vi "DUTDialog.vi"(8 "Error In":errorcluster, 11 "DUT Configuration In":T1={"Count"=1, "Wirings"=[], "Names"=[]}) -> (0 "Error Out":errorcluster, 2 "Cancelled?":bool, 3 "DUT Configuration Out":T1={"Count"=1, "Wirings"=[], "Names"=[]})   [LabVIEW 2012]
uses:
  DUTConfiguration.ctl
  driver/Public/Controls/SMUSense.ctl
  libs/LV-Utilities/LV-Utilities.lvlib
  driver/Keithley-2602.lvlib
panel:
  in  "CANCEL":bool
  in  "DONE":bool
  in  "SMU B Names":string[](array[string])
  in  "SMU B Wiring":enum16{"2-Wire", "4-Wire"}(ring)=enum."4-Wire"
  in  "SMU A Names":string[](array[string])
  in  "SMU A Wiring":enum16{"2-Wire", "4-Wire"}(ring)=enum."4-Wire"
  in  "Count":u32=1 min=1 step=1
  # "Source-Measure Unit A"
  # "Source-Measure Unit B"
  # "Names"
  # "Wiring"
  # "Names"
  # "Wiring"
  # "Number Per SMU:"
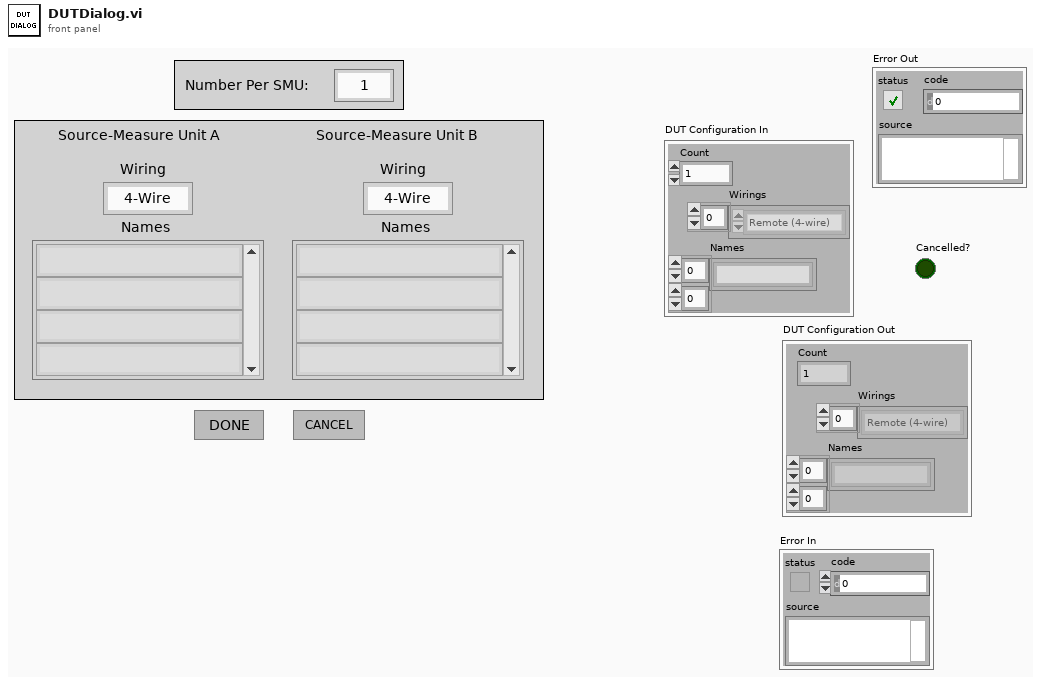
[diagram p1: front panel]
types:
  T1 = typedef "DUTConfiguration.ctl" = cluster{"Count":u32, "Wirings":T2[], "Names":string[][]}
  T2 = typedef "Keithley-2602.lvlib/SMUSense.ctl" = enum16{"Local (2-wire)", "Remote (4-wire)", "Calibration"}
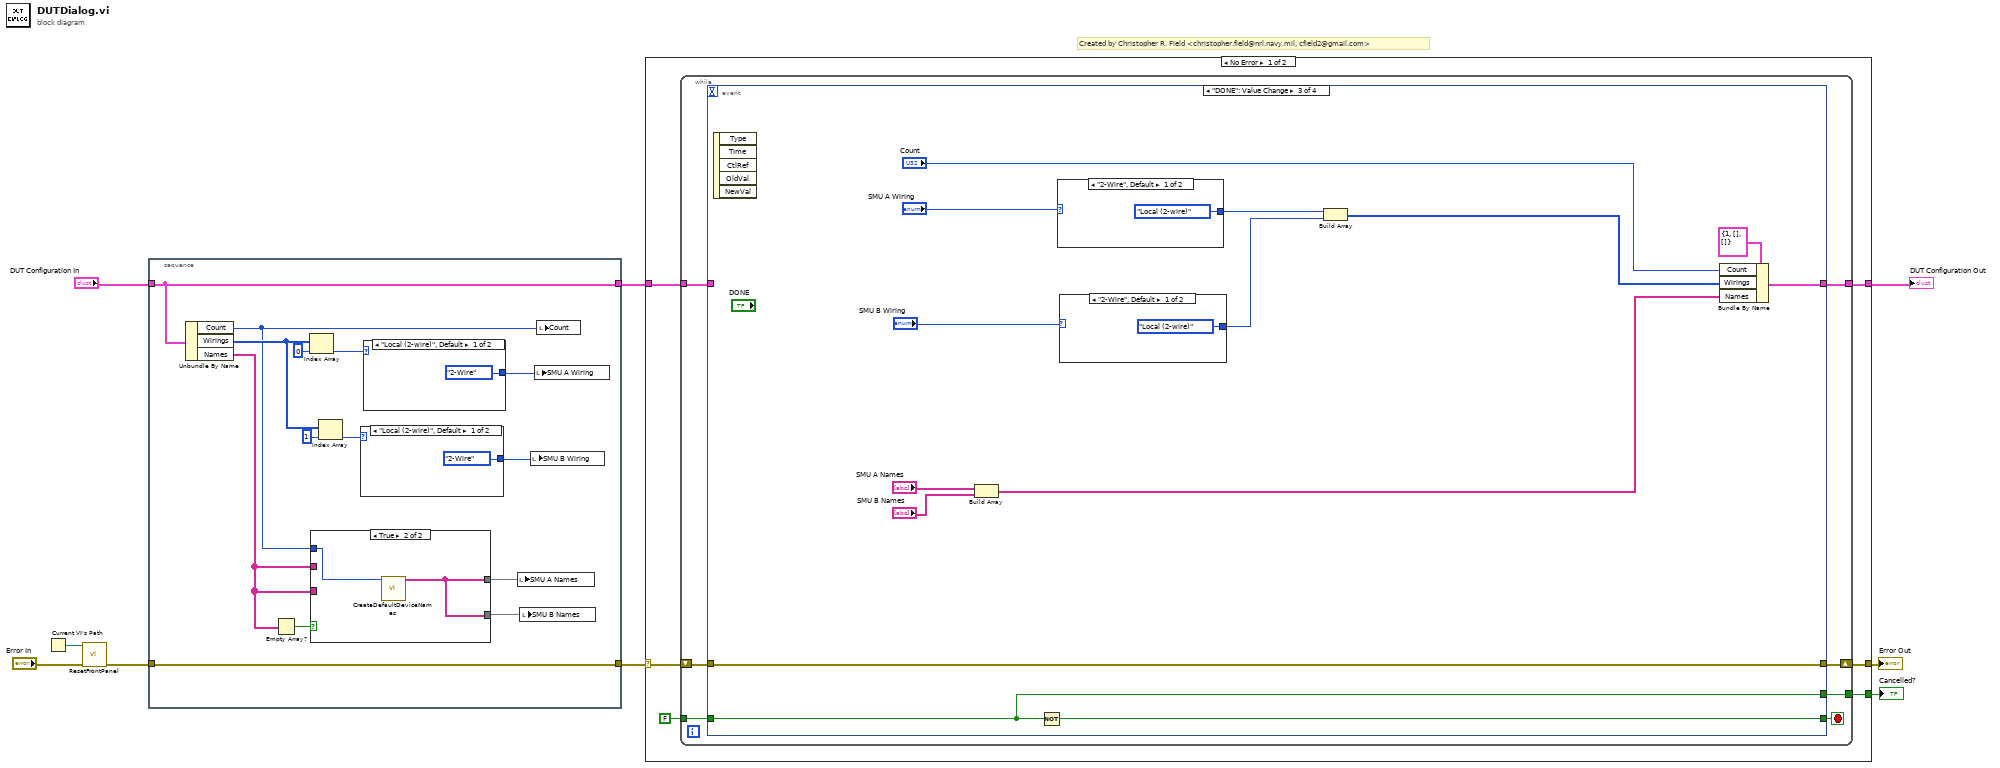
[diagram p0: block diagram]
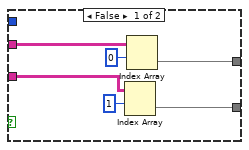
[diagram p2: hidden frame]
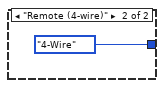
[diagram p3: hidden frame]
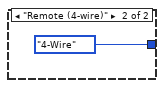
[diagram p4: hidden frame]
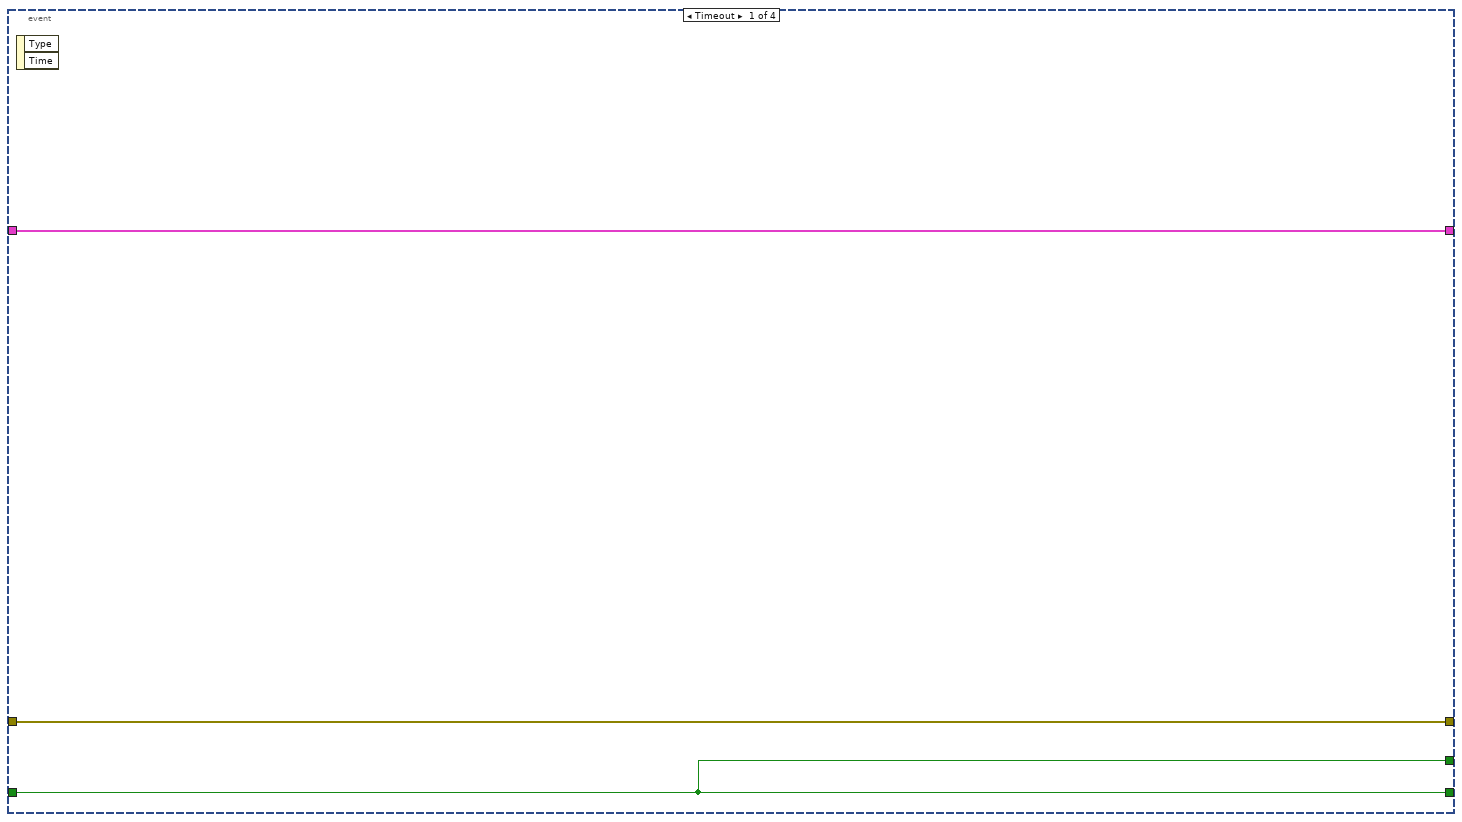
[diagram p5: hidden frame]
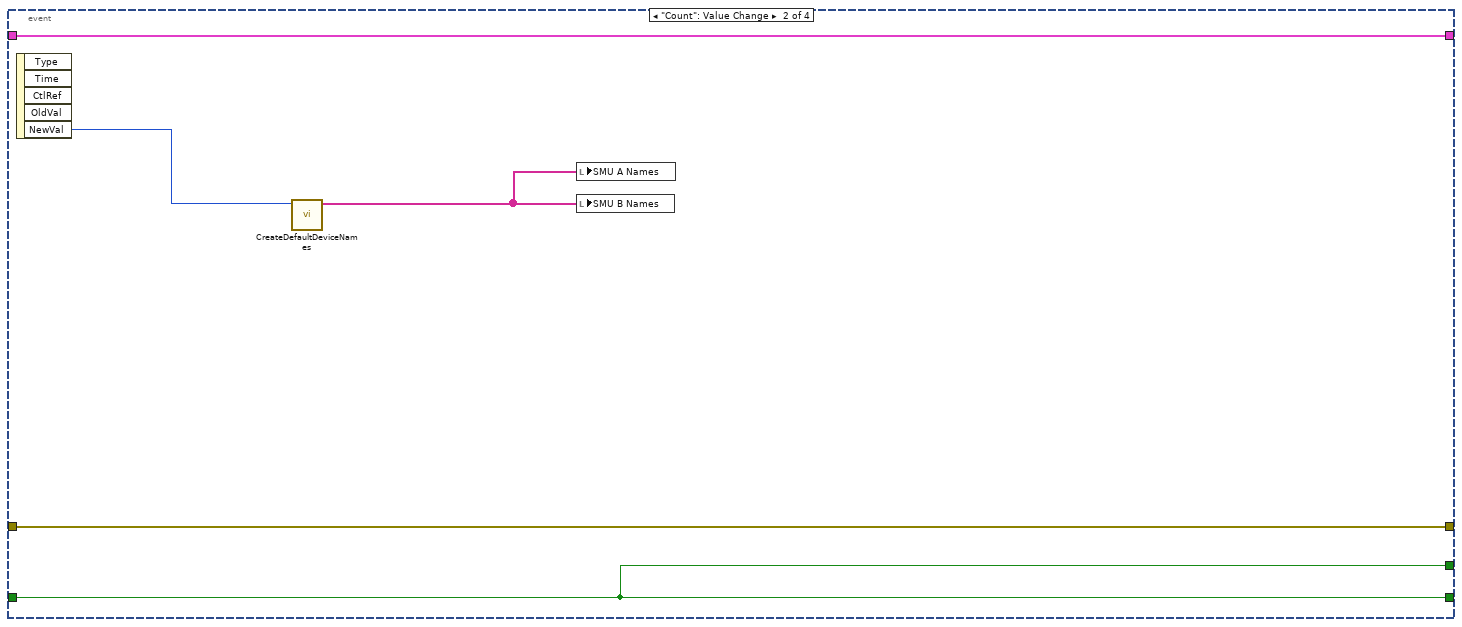
[diagram p6: hidden frame]
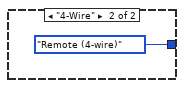
[diagram p7: hidden frame]
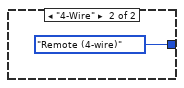
[diagram p8: hidden frame]
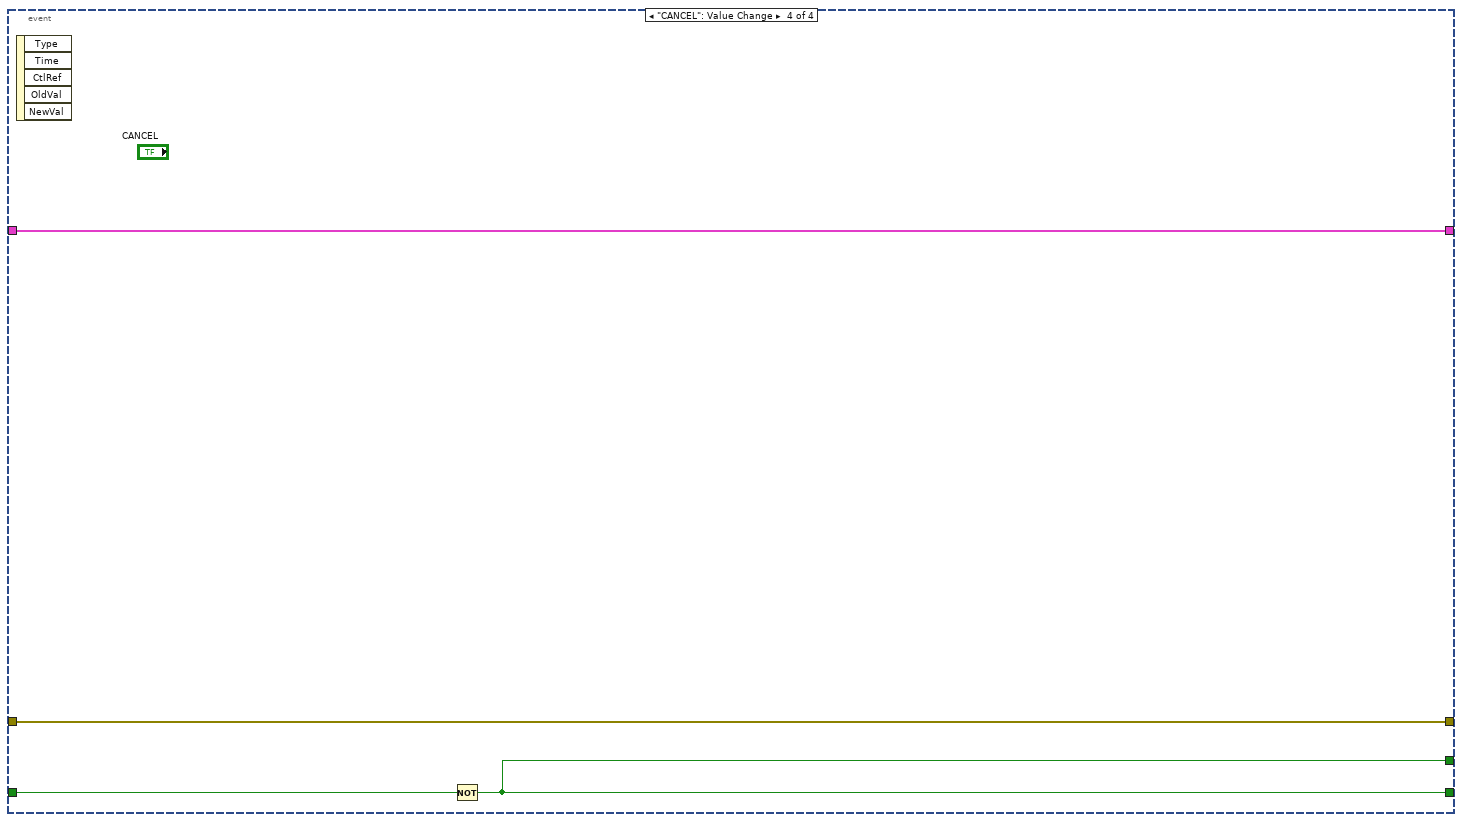
[diagram p9: hidden frame]
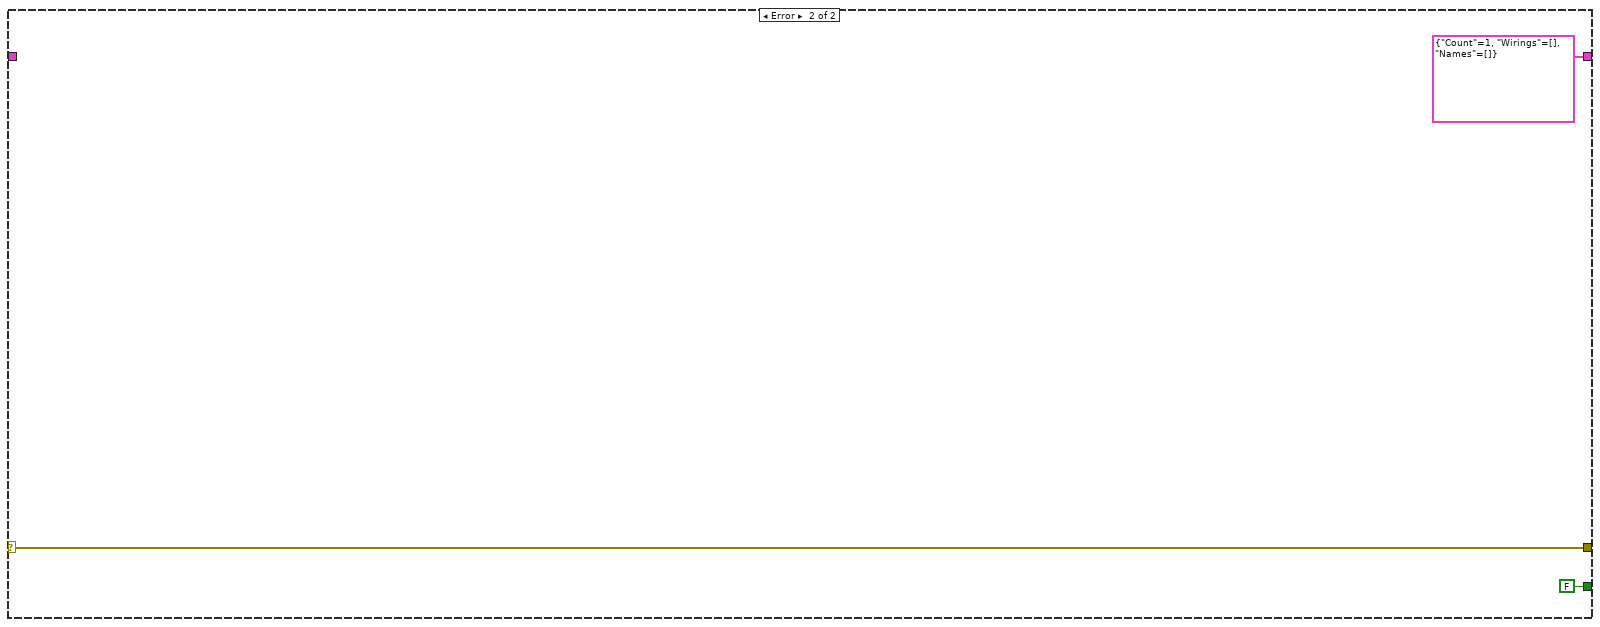
[diagram p10: hidden frame]
diagram:
  # "Created by Christopher R. Field <christopher.field@nrl.navy.mil, cfield2@gmail.com>"
  n1 = Current VI's Path() -> (path=w9:path)
  n2 = call "ResetFrontPanel.vi"("Error In"="Error In", "VI Path"=w9) -> ("Error Out"=w4:errorcluster)  [unwired: 9 in]
  n3 = stacked-sequence {
    tunnel: w4 -> [w23]
    tunnel: [w23] -> w3
    tunnel: "DUT Configuration In" -> [w22]
    tunnel: [w22] -> w1
    frame #0 {
      n4 = Unbundle By Name(w22) -> ("Count"=w10:u32, "Wirings"=w17:T2[], "Names"=w13:string[][])
      n5 = Empty Array?(array=w13) -> (empty?=w14:bool)
      n6 = Index Array(array=w17, index=0) -> (element=w20:T2)
      n7 = case shown="True" w14 {
        tunnel: w13 -> [w27 _]
        tunnel: w13 -> [w26 _]
        tunnel: [w25 w30] -> w12
        tunnel: [w24 w30] -> w11
        tunnel: w10 -> [_ w31]
        frame False {
          n8 = Index Array(array=w26, index (row)=1 ("index")) -> (element=w24:string[])  [unwired: 1 in]
          n9 = Index Array(array=w27, index (row)=0 ("index")) -> (element=w25:string[])  [unwired: 1 in]
        }
        frame True {
          n10 = call "CreateDefaultDeviceNames.vi"("DUT Count"=w31) -> ("Default Device Names"=w30:string[])  [unwired: 10 in]
        }
      }
      n11 = Index Array(array=w17, index=1) -> (element=w16:T2)
      n12 = case shown="\"Local (2-wire)\", Default" w16 {
        tunnel: [enum16{"2-Wire", "4-Wire"}."2-Wire" ("SMU A Wiring") enum16{"2-Wire", "4-Wire"}."4-Wire" ("SMU A Wiring")] -> w15
        frame "Local (2-wire)", Default {
        }
        frame "Remote (4-wire)" {
        }
      }
      n13 = case shown="\"Local (2-wire)\", Default" w20 {
        tunnel: [enum16{"2-Wire", "4-Wire"}."2-Wire" ("SMU A Wiring") enum16{"2-Wire", "4-Wire"}."4-Wire" ("SMU A Wiring")] -> w19
        frame "Local (2-wire)", Default {
        }
        frame "Remote (4-wire)" {
        }
      }
      n14 = local write "SMU A Names"(w12) -> ()
      n15 = local write "SMU B Names"(w11) -> ()
      n16 = local write "SMU B Wiring"(w15) -> ()
      n17 = local write "SMU A Wiring"(w19) -> ()
      n18 = local write "Count"(w10) -> ()
    }
  }
  n19 = case shown="No Error" w3 {
    selector: w3 -> [w41 w81]
    tunnel: [w40 w81] -> w7
    tunnel: [w38 FALSE] -> w6
    tunnel: [w37 T1 {"Count"=1, "Wirings"=[], "Names"=[]} ("DUT Configuration")] -> w5
    tunnel: w1 -> [w36 _]
    frame No Error {
      n20 = while {
        shift-right: [w47] -> w40
        shift-left: w41 -> [w48]
        tunnel: FALSE -> [w46]
        tunnel: [w44] -> w38
        tunnel: w36 -> [w42]
        tunnel: [w43] -> w37
        stop <- w45 stop-if-true
        n21 = event shown="[2] \"DONE\": Value Change" {
          selector: _ -> [_ _ _ _]
          dyn-events: _ -> [_ _ _ _]
          timeout: _ -> [_ _ _ _]
          tunnel: w48 -> [w51 w56 w70 w77]
          tunnel: [w51 w56 w70 w77] -> w47
          tunnel: w46 -> [w50 w55 w68 w76]
          tunnel: [w50 w55 w69 w75] -> w45
          tunnel: [w50 w55 w68 w75] -> w44
          tunnel: [w49 w54 w62 w78] -> w43
          tunnel: w42 -> [w49 w54 _ w78]
          event Timeout {
            n22 = event-data() -> ()  [unwired: 1 in, 2 out]
          }
          event "Count": Value Change {
            n23 = event-data() -> ("NewVal"=w53:u32)  [unwired: 1 in, 4 out]
            n24 = call "CreateDefaultDeviceNames.vi"("DUT Count"=w53) -> ("Default Device Names"=w52:string[])  [unwired: 10 in]
            n25 = local write "SMU A Names"(w52) -> ()
            n26 = local write "SMU B Names"(w52) -> ()
          }
          event "DONE": Value Change {
            n27 = event-data() -> ()  [unwired: 1 in, 5 out]
            n28 = Build Array("SMU A Names", "SMU B Names") -> (w63:string[][])
            n29 = Not(x=w68) -> (.not. x?=w69:bool)
            n30 = case shown="\"2-Wire\", Default" "SMU A Wiring" {
              tunnel: [SMUSense."Local (2-wire)" ("SMU Sense") SMUSense."Remote (4-wire)" ("SMU Sense")] -> w59
              frame "2-Wire", Default {
              }
              frame "4-Wire" {
              }
            }
            n31 = case shown="\"2-Wire\", Default" "SMU B Wiring" {
              tunnel: [SMUSense."Local (2-wire)" ("SMU Sense") SMUSense."Remote (4-wire)" ("SMU Sense")] -> w58
              frame "2-Wire", Default {
              }
              frame "4-Wire" {
              }
            }
            n32 = Build Array(w59, w58) -> (w57:T2[])
            n33 = Bundle By Name(cluster=T1 {"Count"=1, "Wirings"=[], "Names"=[]} ("DUT Configuration"), "Count"="Count", "Wirings"=w57, "Names"=w63) -> (w62:T1)
          }
          event "CANCEL": Value Change {
            n34 = event-data() -> ()  [unwired: 1 in, 5 out]
            n35 = Not(x=w76) -> (.not. x?=w75:bool)
          }
        }
      }
    }
    frame Error {
    }
  }
  "Cancelled?" <- w6
  "DUT Configuration Out" <- w5
  "Error Out" <- w7
